vi "Process.vi"(8 "error in":errorcluster, 11 "TestDefaultDirectory In":refnum<class "Maui.Test.DefaultDirectory.lvclass">) -> (0 "error out":errorcluster, 3 "TestDefaultDirectory Out":refnum<class "Maui.Test.DefaultDirectory.lvclass">)   [LabVIEW 2019, in "Maui.Test.DefaultDirectory.lvclass"]
doc: "---------------------------------------------------------------\nJKI State Machine Objects™\nhttp://jki.net/state-machine-objects/\nCopyright (C) 2005-2015, JKI <info@jki.net>\nALL RIGHTS RESERVEDJKI State Machine Objects (SMO) 1.0.0.5\nJKI - JKI\nCopyright (c) 2016, JKI"
uses:
  Maui.Test.DefaultDirectory.lvclass
  C:/Program Files (x86)/National Instruments/LabVIEW 2019/vi.lib/JKI/JKI SMO/SMO/SMO.lvclass
  C:/Users/patrick/Documents/GitHub/MAUI-Engine/lvsrc/Maui 1.0/SMO.UI.MAUI/MAUI.lvclass
  C:/Program Files (x86)/National Instruments/LabVIEW 2019/vi.lib/JKI/JKI SMO/SMO.UI/SMO.UI.lvclass
  <vilib>/JKI/JKI SMO/SMO/Typedefs/Parent Call--Enum.ctl
  <userlib>/LevyLab/Embedded UI/SMO.UI.Embedded/Embedded UI.lvclass
  <vilib>/JKI/JKI SMO/SMO/SMO.lvclass/SMO.ctl
  Maui.Test.DefaultDirectory.lvclass/Maui.Test.DefaultDirectory.ctl
  lvsrc/Maui 1.0/SMO.UI.MAUI/Typedefs/PanelData.ctl
  <vilib>/JKI/JKI SMO/SMO/Private/ReftoDVR--SMO.vi
  <vilib>/addons/_JKI Toolkits/Caraya/classes/Assert/Assert True.vi
  <vilib>/addons/_JKI Toolkits/Caraya/classes/Assert/Assert Equal Value_Variant.vi
  lvsrc/Maui 1.0/SMO.UI.MAUI/MAUI.lvclass
  <vilib>/JKI/JKI SMO/SMO/SMO.lvclass
  <vilib>/JKI/JKI SMO/SMO.UI/SMO.UI.lvclass
  <vilib>/addons/_JKI Toolkits/Caraya/classes/Test/Test.lvclass
  <vilib>/addons/_JKI Toolkits/Caraya/classes/Assert/Assert.lvclass
panel:
  in  "Ring 2":u16(ring)
  in  "Ring 1":u16(ring)
  # "For instructions on how to use the JKI State Machine Objects, examples and video tutorials, visit:\nhttp://jki.net/state-machine-objects/\n\nJKI State Machine Objects™\nhttp://jki.net/state-machine-objects/\nCopyright (C) 2005-2015, JKI <info@jki.net>\nALL RIGHTS RESERVED"
  # "Test Default Directory"
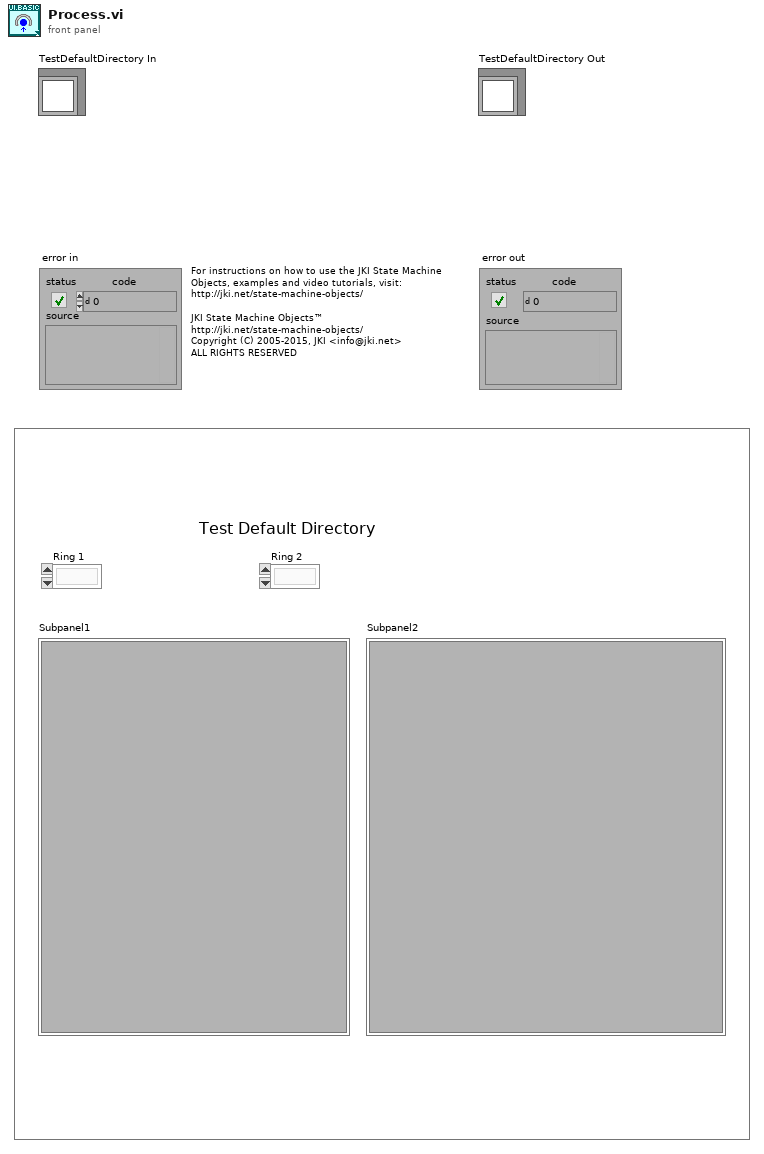
[diagram p1: front panel]
types:
  T1 = typedef "SMO.lvclass/Parent Call--Enum.ctl" = enum16{"Allows parent to run", "Does not request parent to run"}
  T2 = enum32{"invalid app kind", "Development System", "Run Time System", "Student Edition", "Embedded LabVIEW", "Evaluation", "Custom"}
  T3 = enum32{"Invalid", "Standard", "Closed", "Hidden", "Minimized", "Maximized"}
  T4 = cluster{"Core":cluster{"Current VI Reference":refnum<vi>, "Close Panel on Exit?":bool, "error":errorcluster}, "Self Reference":refnum<class "Maui.Test.DefaultDirectory.lvclass">, "Subpanel1":refnum<vi>, "Subpanel2":refnum<vi>, "Ring 1":refnum<vi>, "Ring 2":refnum<vi>, "Subpanels":refnum<class "Embedded UI.lvclass">[]}
  T5 = cluster{"Current VI Reference":refnum<vi>, "Close Panel on Exit?":bool, "error":errorcluster}
  T6 = typedef "SMO.lvclass/Protected Events.ctl" = cluster{"StopProcesses":refnum<user-event>, "AbortProcesses":refnum<user-event>, "Config Changed":refnum<user-event>, "Dependency":refnum<user-event>}
  T7 = typedef "MAUI.lvclass/PublicEvents--Cluster.ctl" = cluster{"ReadyForInfo ":refnum<user-event>}
  T8 = typedef "MAUI.lvclass/PanelData.ctl" = cluster{"SubPanel":refnum<vi>, "Ring":refnum<vi>, "Active":i32}
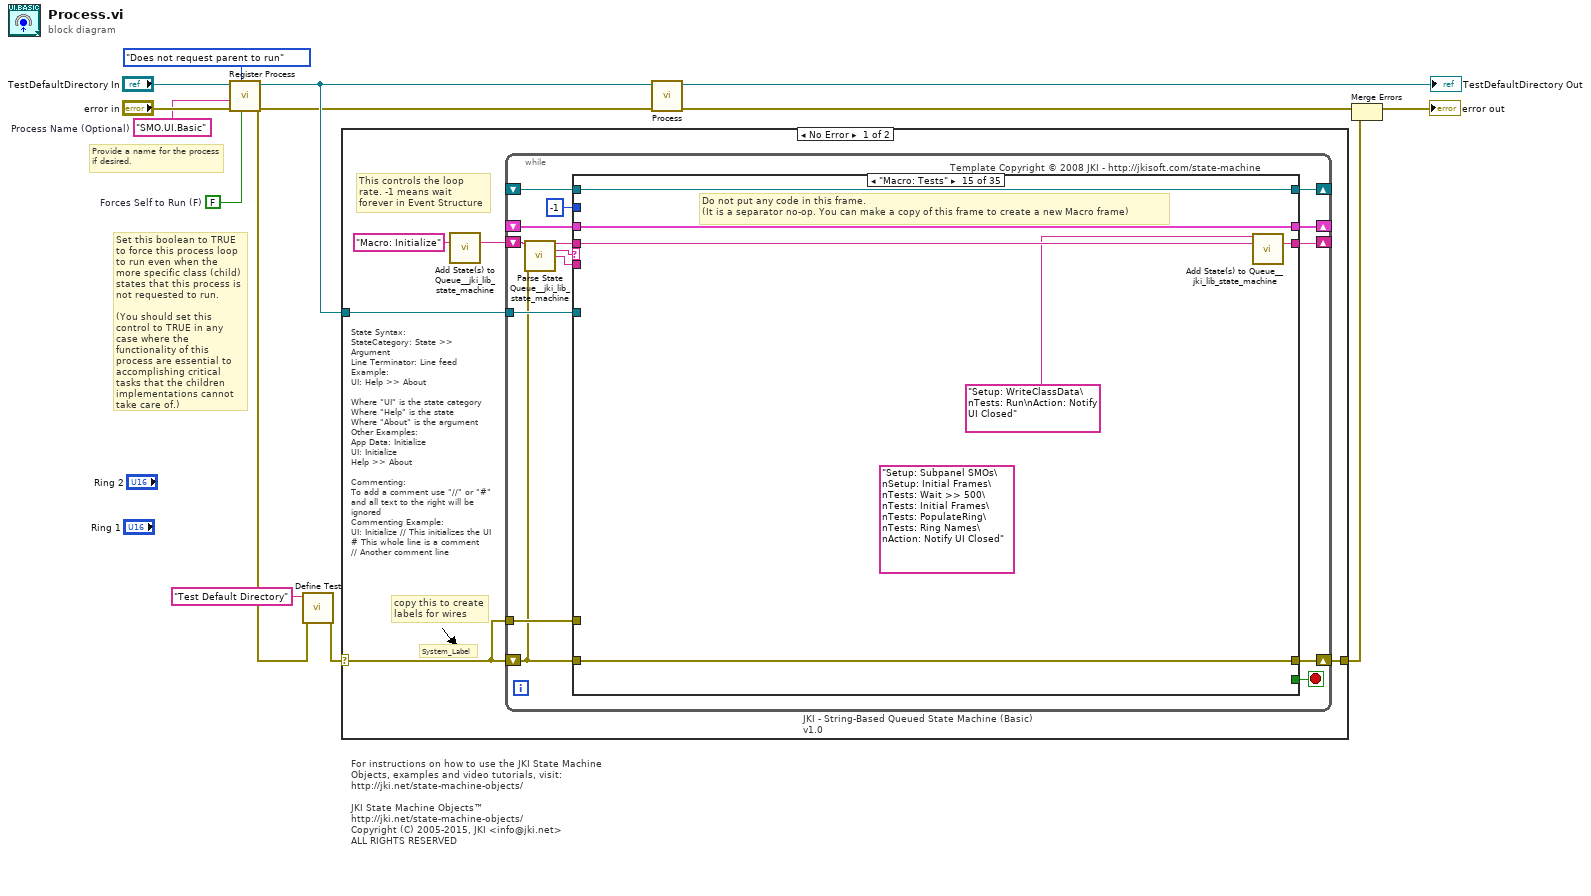
[diagram p0: block diagram]
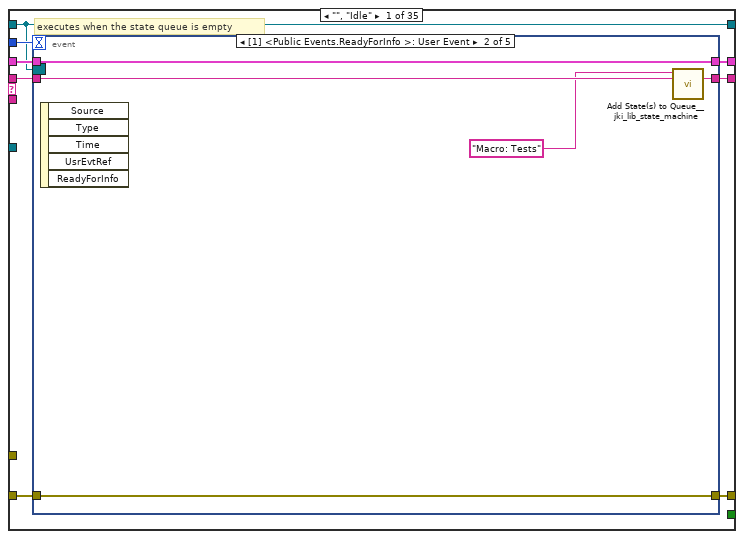
[diagram p2: hidden frame]
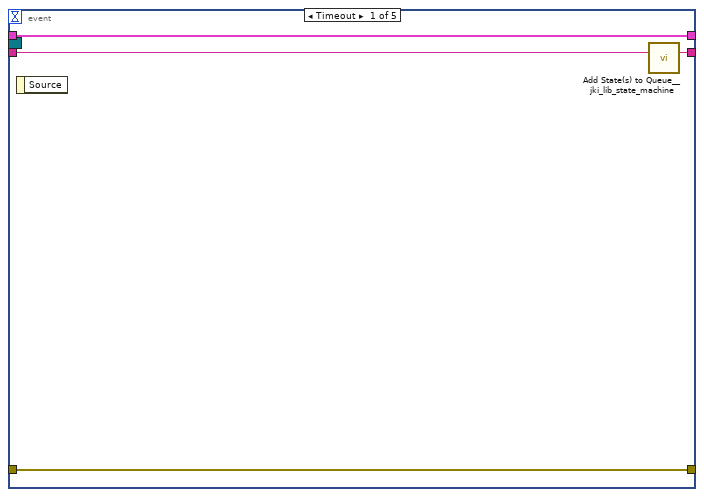
[diagram p3: hidden frame]
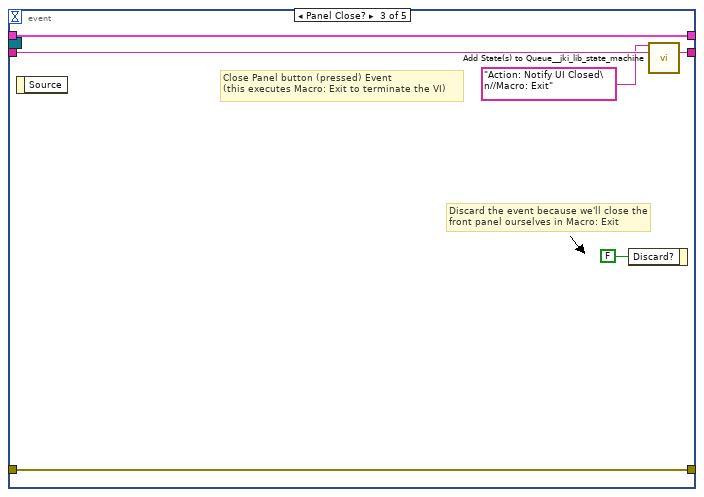
[diagram p4: hidden frame]
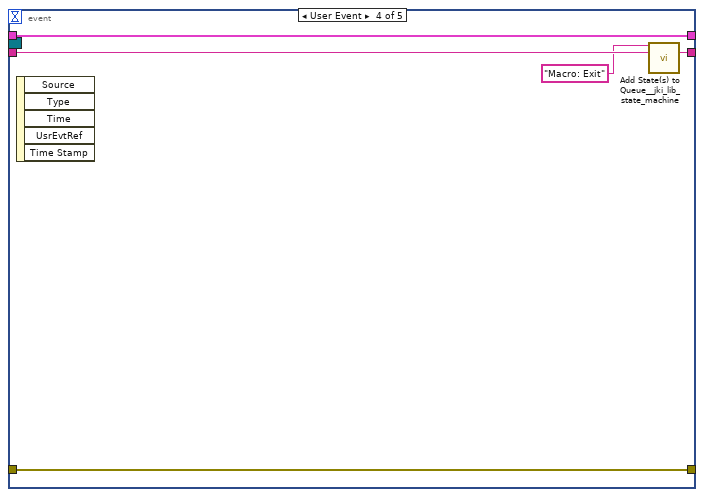
[diagram p5: hidden frame]
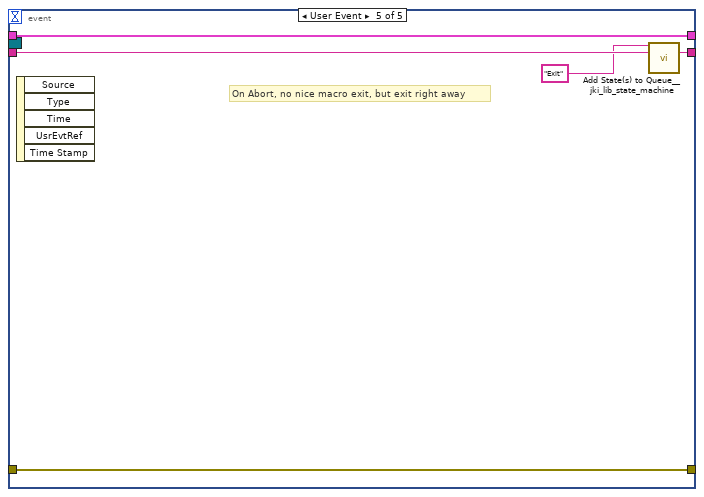
[diagram p6: hidden frame]
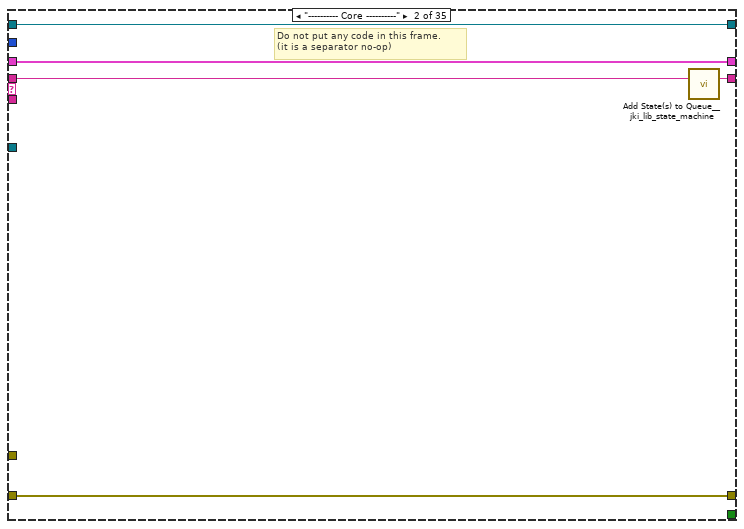
[diagram p7: hidden frame]
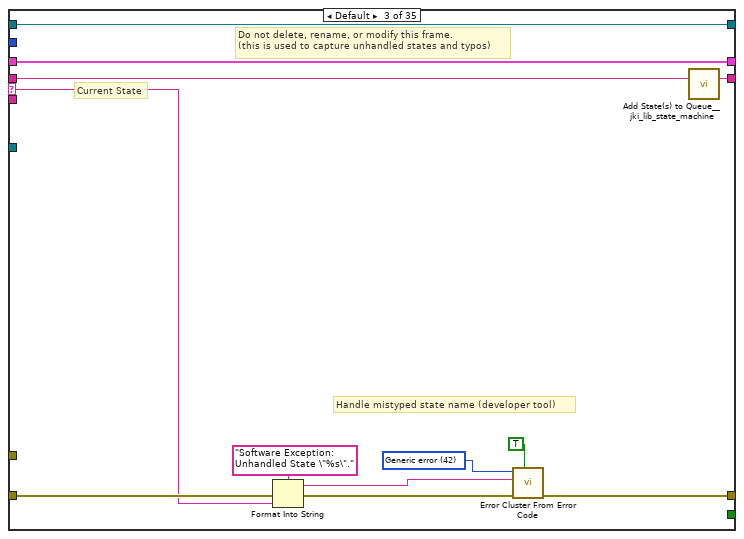
[diagram p8: hidden frame]
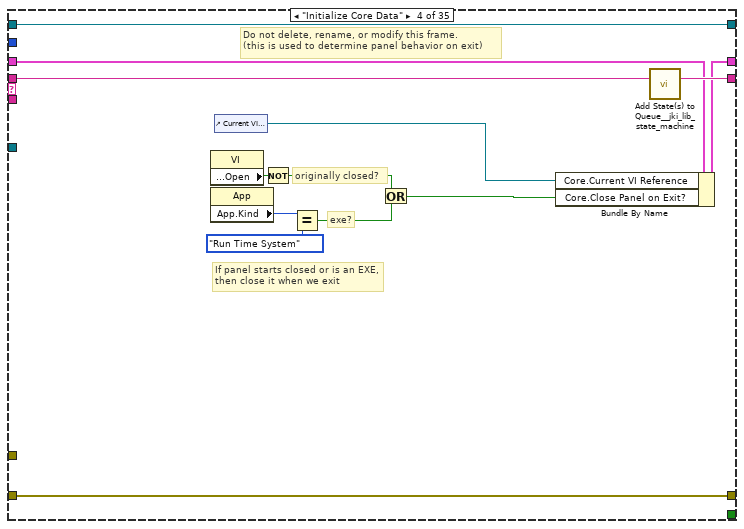
[diagram p9: hidden frame]
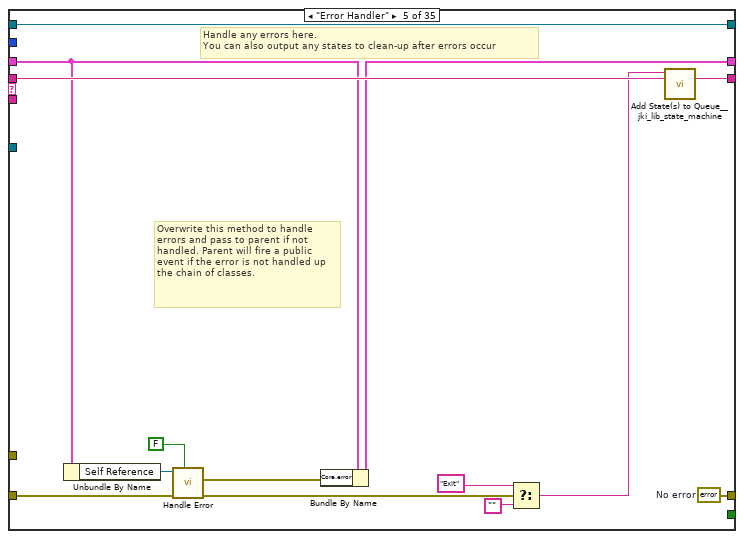
[diagram p10: hidden frame]
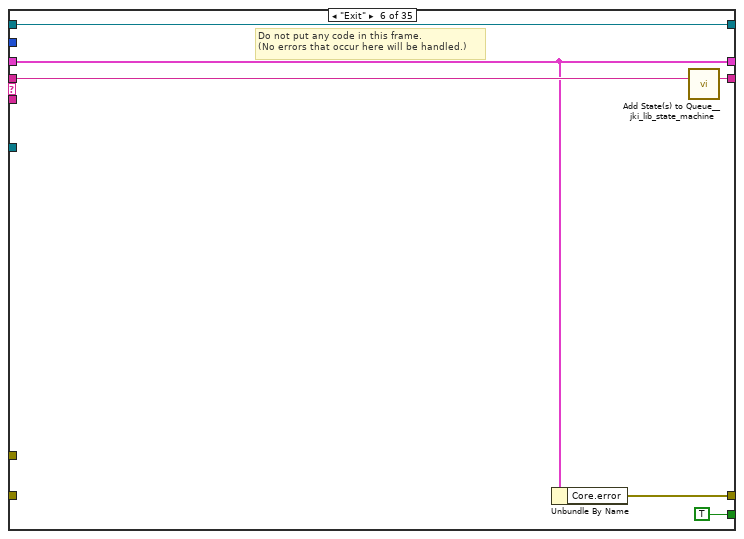
[diagram p11: hidden frame]
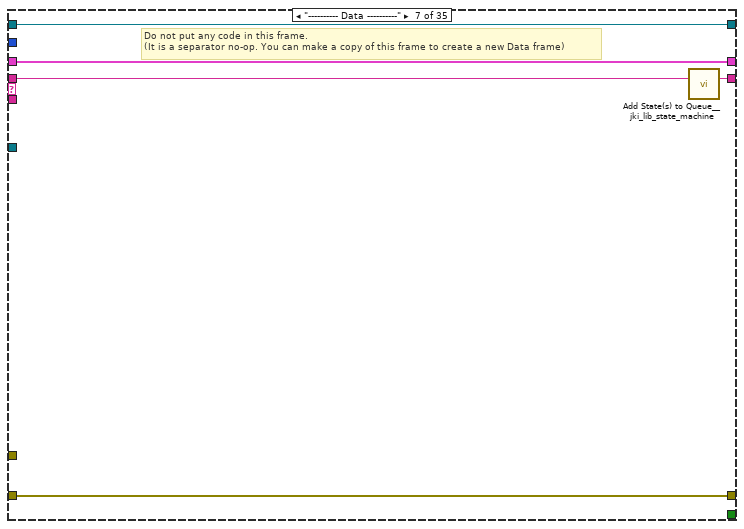
[diagram p12: hidden frame]
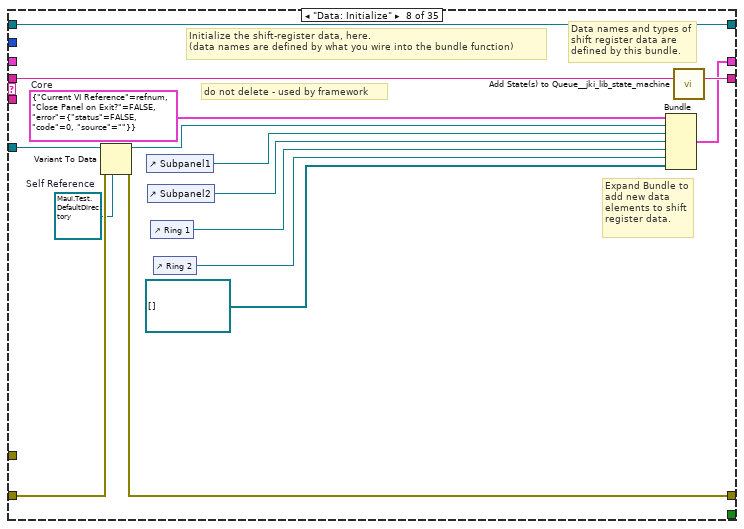
[diagram p13: hidden frame]
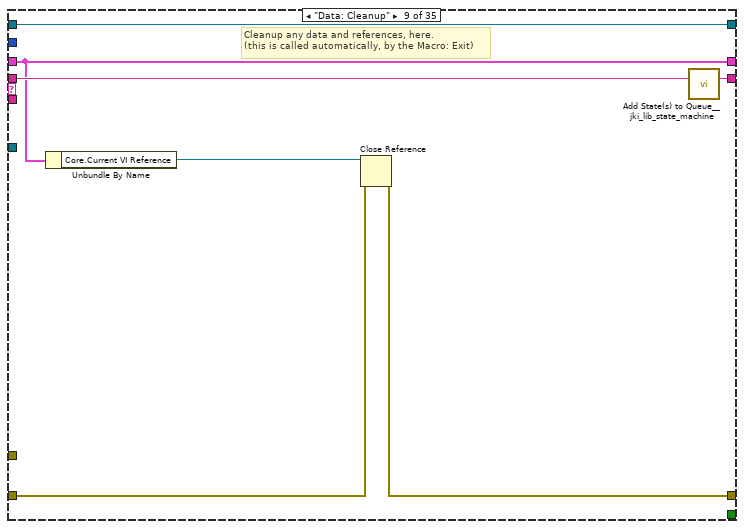
[diagram p14: hidden frame]
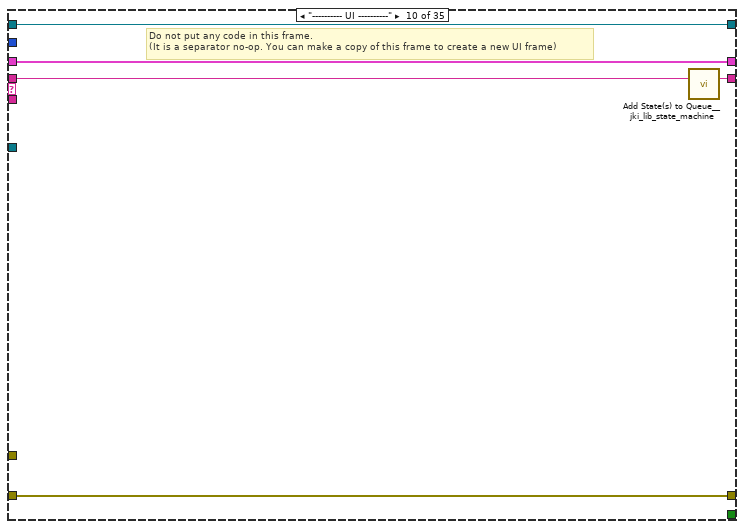
[diagram p15: hidden frame]
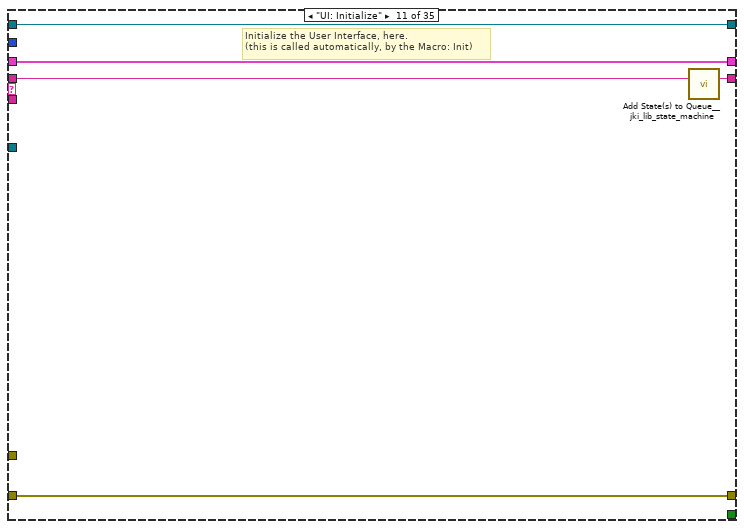
[diagram p16: hidden frame]
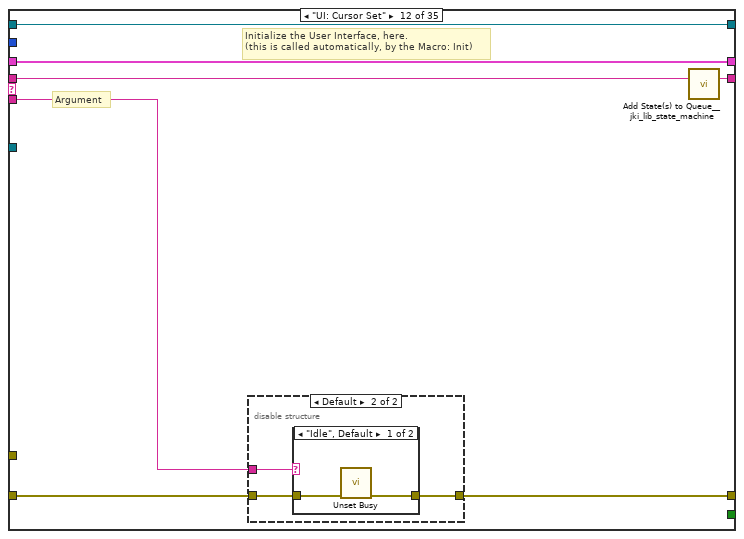
[diagram p17: hidden frame]
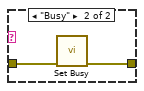
[diagram p19: hidden frame]
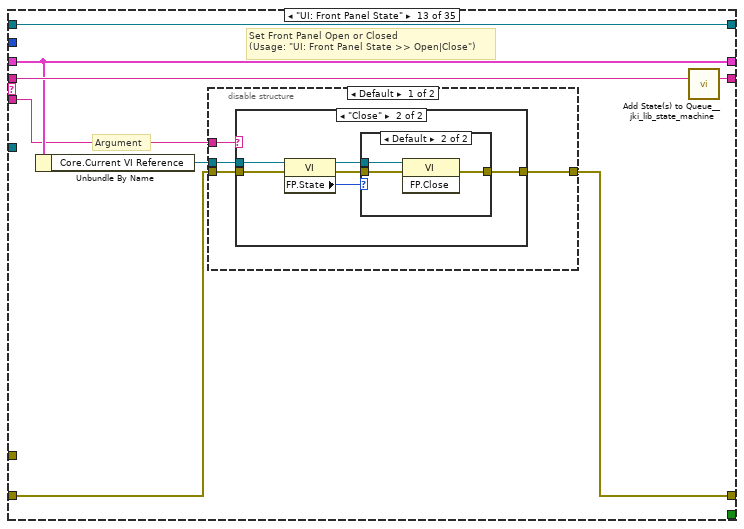
[diagram p20: hidden frame]
diagram:
  w5 = FALSE  # Forces Self to Run (F)
  w4 = "SMO.UI.Basic"  # Process Name (Optional)
  # "Provide a name for the process\nif desired."
  # "Set this boolean to TRUE to force this process loop to run even when the more specific class (child) states that this process is not requested to run.\n\n(You should set this control to TRUE in any case where the functionality of this process are essential to accomplishing critical tasks that the children implementations cannot take care of.)"
  # "For instructions on how to use the JKI State Machine Objects, examples and video tutorials, visit:\nhttp://jki.net/state-machine-objects/\n\nJKI State Machine Objects™\nhttp://jki.net/state-machine-objects/\nCopyright (C) 2005-2015, JKI <info@jki.net>\nALL RIGHTS RESERVED"
  n1 = call <vilib>:"Register Process.vi"("Forces Self to Run (F)"=w5, "Parent Call"=Parent_Call--Enum."Does not request parent to run", "error in (no error)"="error in", "Process Name (optional)"=w4, "SMO"="TestDefaultDirectory In") -> ("error out"=w3:errorcluster, "SMO out"=w10:refnum<class "Maui.Test.DefaultDirectory.lvclass">)  [unwired: 5 in]
  n2 = call <vilib>:"Define Test.vi"("error in (no error)"=w3, "Label (VI Title)"="Test Default Directory") -> ("error out"=w2:errorcluster)  [unwired: 9 in]
  n3 = case shown="No Error" w2 {
    selector: w2 -> [w15 w466]
    tunnel: w10 -> [w16 _]
    tunnel: [w14 w466] -> w7
    frame No Error {
      # "State Syntax:\nStateCategory: State >> Argument\nLine Terminator: Line feed\nExample:\nUI: Help >> About\n\nWhere \"UI\" is the state category\nWhere \"Help\" is the state\nWhere \"About\" is the argument\nOther Examples:\nApp Data: Initialize\nUI: Initialize\nHelp >> About\n\nCommenting:\nTo add a comment use \"//\" or \"#\" and all text to the right will be ignored\nCommenting Example:\nUI: Initialize // This initializes the UI\n# This whole line is a comment\n// Another comment line"
      # "copy this to create labels for wires"
      # "This controls the loop rate. -1 means wait forever in Event Structure"
      # "System_Label"
      n4 = call <vilib>:"Add State(s) to Queue__jki_lib_state_machine.vi"("State(s) in (\"\")"="Macro: Initialize") -> ("States Out"=w17:string)  [unwired: 14 in]
      n5 = while "JKI - String-Based Queued State Machine (Basic) v1.0" {
        shift-right: [w26] -> _
        shift-left: _ -> [w25]
        shift-right: [w29] -> w14
        shift-left: w15 -> [w19]
        shift-right: [w28] -> _
        shift-left: w17 -> [w30]
        tunnel: w16 -> [w23]
        shift-right: [w22] -> _
        shift-left: _ -> [w21]
        tunnel: w15 -> [w20]
        stop <- w27 stop-if-true
        # "Template Copyright © 2008 JKI - http://jkisoft.com/state-machine"
        n6 = call <vilib>:"Parse State Queue__jki_lib_state_machine.vi"("State Queue"=w30, "Error In (no error)"=w19) -> ("Remaining States"=w32:string, "Current State"=w33:string, "Arguments"=w31:string)  [unwired: 11 in]
        n7 = case shown="\"Macro: Tests\"" w33 {
          selector: w33 -> [_ _ w73 _ _ _ _ _ _ _ _ _ _ _ _ _ _ _ _ _ _ _ _ _ _ _ _ _ _ _ _ _ _ _ _]
          tunnel: w32 -> [w41 w71 w77 w96 w110 w116 w121 w136 w143 w148 w153 w160 w176 w208 w214 w223 w237 w242 w253 w258 w270 w276 w283 w290 w297 w309 w319 w338 w345 w359 w369 w398 w407 w427 w465]
          tunnel: w31 -> [_ _ _ _ _ _ _ _ _ _ _ w154 w170 _ _ _ _ _ _ _ _ _ _ _ _ _ _ _ _ _ _ _ w402 _ _]
          tunnel: w25 -> [w39 w68 w75 w87 w99 w112 w118 _ w138 w145 w151 w158 w172 w205 w211 w219 w228 w239 w250 w255 w268 w274 w279 w286 w293 w305 w316 w335 w341 w356 w366 w395 w403 w420 w460]
          tunnel: [w38 w69 w79 w93 w101 w111 w119 w132 w139 w146 w150 w155 w173 w206 w212 w221 w235 w240 w244 w256 w263 w271 w280 w284 w294 w306 w312 w331 w342 w347 w364 w390 w404 w421 w446] -> w29
          tunnel: w19 -> [w37 w69 w78 w93 w106 _ w119 w133 w140 w146 w150 w156 w174 w206 w212 w221 w235 w240 w245 w256 w265 w272 w280 w285 w294 w306 w311 w330 w342 w349 w362 w376 w400 w409 w445]
          tunnel: [w40 w70 w76 w95 w109 w115 w120 w135 w142 w147 w152 w159 w175 w207 w213 w222 w236 w241 w252 w257 w269 w275 w282 w289 w296 w308 w318 w337 w344 w358 w368 w397 w406 w426 w464] -> w28
          tunnel: [_ _ _ _ _ TRUE _ _ _ _ _ _ _ _ _ _ _ _ _ _ _ _ _ _ _ _ _ _ _ _ _ _ _ _ _] -> w27
          tunnel: [w36 w68 w75 w94 w98 w112 w118 w134 w138 w145 w151 w158 w172 w205 w211 w219 w228 w239 w250 w255 w268 w274 w278 w286 w292 w304 w315 w334 w340 w355 w365 w394 w403 w420 w460] -> w26
          tunnel: -1 ("Timeout") -> [w35 _ _ _ _ _ _ _ _ _ _ _ _ _ _ _ _ _ _ _ _ _ _ _ _ _ _ _ _ _ _ _ _ _ _]
          tunnel: w23 -> [_ _ _ _ _ _ _ w131 _ _ _ _ _ _ _ _ _ _ _ _ _ _ _ _ _ _ _ _ _ _ _ _ _ _ _]
          tunnel: [w34 w67 w72 w84 w108 w113 w117 w129 w137 w144 w149 w157 w169 w204 w210 w220 w229 w238 w251 w254 w267 w273 w281 w288 w295 w307 w317 w336 w343 w357 w367 w396 w405 w425 w463] -> w22
          tunnel: w21 -> [w34 w67 w72 w84 w108 w113 w117 w129 w137 w144 w149 w157 w169 w204 w210 w220 w229 w238 w251 w254 _ w273 w281 w288 w295 w307 w317 w336 w343 w357 w367 w396 w405 w425 w463]
          tunnel: w20 -> [_ _ _ _ _ _ _ _ _ _ _ _ _ _ _ _ _ _ _ _ _ _ _ _ _ _ _ _ _ w346 _ w375 _ w408 w431]
          frame "", "Idle" {
            # "executes when the state queue is empty"
            n8 = event shown="[1] <Public Events.ReadyForInfo >: User Event" {
              selector: w34 -> [_ _ _ _ _]
              dyn-events: _ -> [_ _ _ _ _]
              timeout: w35 -> [_ _ _ _ _]
              tunnel: w41 -> [w45 w50 w56 w61 w66]
              tunnel: [w44 w49 w55 w60 w65] -> w40
              tunnel: w39 -> [w42 w47 w52 w58 w63]
              tunnel: [w43 w48 w51 w59 w64] -> w38
              tunnel: w37 -> [w43 w48 w51 w59 w64]
              tunnel: [w42 w47 w52 w58 w63] -> w36
              event Timeout {
                n9 = event-data() -> ()  [unwired: 1 in, 1 out]
                n10 = call <vilib>:"Add State(s) to Queue__jki_lib_state_machine.vi"("State(s) in (\"\")"=w45) -> ("States Out"=w44:string)  [unwired: 14 in]
              }
              event User Event {
                n11 = event-data() -> ()  [unwired: 1 in, 5 out]
                n12 = call <vilib>:"Add State(s) to Queue__jki_lib_state_machine.vi"("State(s) in Front (\"\")"="Macro: Tests", "State(s) in (\"\")"=w50) -> ("States Out"=w49:string)  [unwired: 13 in]
              }
              event Panel Close? {
                # "Discard the event because we'll close the front panel ourselves in Macro: Exit"
                # "Close Panel button (pressed) Event\n(this executes Macro: Exit to terminate the VI)"
                n13 = event-data() -> ()  [unwired: 1 in, 1 out]
                n14 = event-data ("Event Filter Node")("Discard?"=FALSE) -> ()  [unwired: 1 in, 1 out]
                n15 = call <vilib>:"Add State(s) to Queue__jki_lib_state_machine.vi"("State(s) in Front (\"\")"="Action: Notify UI Closed\n//Macro: Exit", "State(s) in (\"\")"=w56) -> ("States Out"=w55:string)  [unwired: 13 in]
              }
              event User Event {
                n16 = event-data() -> ()  [unwired: 1 in, 5 out]
                n17 = call <vilib>:"Add State(s) to Queue__jki_lib_state_machine.vi"("State(s) in Front (\"\")"="Macro: Exit", "State(s) in (\"\")"=w61) -> ("States Out"=w60:string)  [unwired: 13 in]
              }
              event User Event {
                # "On Abort, no nice macro exit, but exit right away"
                n18 = event-data() -> ()  [unwired: 1 in, 5 out]
                n19 = call <vilib>:"Add State(s) to Queue__jki_lib_state_machine.vi"("State(s) in Front (\"\")"="Exit", "State(s) in (\"\")"=w66) -> ("States Out"=w65:string)  [unwired: 13 in]
              }
            }
          }
          frame "---------- Core ----------" {
            # "Do not put any code in this frame.\n(it is a separator no-op)"
            n20 = call <vilib>:"Add State(s) to Queue__jki_lib_state_machine.vi"("State(s) in (\"\")"=w71) -> ("States Out"=w70:string)  [unwired: 14 in]
          }
          frame Default {
            w82 = 42 items=["No error", "Argument error", "Memory is full", "Out of zone", "End of file", "File already open", "Generic file I/O error", "File not found", "File permission error", "Disk is full", "Duplicate path", "Too many files open", "System feature not enabled", "Resource file not found", "Cannot add resource", "Resource not found", "Image not found", "Image memory error", "Pen does not exist", "Config type invalid", "Config token not found", "Config parse error", "Config memory error", "Bad external code format", "Bad external code offset", "External code not present", "Null window", "Destroy window error", "Null menu", "Print aborted", "Bad print record", "Print driver error", "Windows error during printing", "Memory error during printing", "Print dialog error", "Generic print error", "Invalid device refnum", "Device not found", "Device parameter error", "Device unit error", "Cannot open device", "Device call aborted", "Generic error", "Cancelled by user", "Object ID too low", "Object ID too high", "Object not in heap", "Unknown heap", "Unknown object (invalid DefProc)", "Unknown object (DefProc not in table)", "Message out of range", "Invalid (null) method", "Unknown message", "Manager call not supported", "Bad address", "Network operation in progress", "Network operation timed out", "Connection is busy", "Network attribute not supported", "Network error", "Address in use", "System out of memory", "Connection aborted", "Connection refused", "Not connected", "Already connected", "Connection closed", "Initialization error (interapplication manager)", "Bad occurrence", "Wait on unbound occurrence handler", "Occurrence queue overflow", "Datalog type conflict", "Unused", "Unrecognized type (interapplication manager)", "Memory corrupt", "Failed to make temporary DLL", "Old CIN version", "Drag socket not found", "Failed to load drop-object", "Failed to register OLE object", "Failed to release OLE object", "Format specifier type mismatch", "Unknown format specifier", "Too few format specifiers", "Too many format specifiers", "Scan failed", "Newer CIN version", "Error converting to variant", "Runtime menu error", "Password tampered", "Variant attribute not found", "Incompatible variant data type", "Event data is not available", "Event Store is not present", "Occurrence is not found", "Event Queue is not created", "Event info is not available", "Refnum passed is NULL", "Error retrieving Class GUID", "Error retrieving CoClass GUID", "Error retrieving TypeLib GUID.", "Bad built application magic bytes.", "Specific driver is different from the specific driver associated with the Logical Name.", "There is no session opened to the class driver.", "Max Error", "MAX - Error with config objects", "MAX - Error loading configuration", "MAX - Group not supported"]
            # "Current State"
            # "Do not delete, rename, or modify this frame.\n(this is used to capture unhandled states and typos)"
            # "Handle mistyped state name (developer tool)"
            n21 = Format Into String(format string="Software Exception: Unhandled State \"%s\"." ("message"), error in=w78, w73) -> (resulting string=w81:string, error out=w80:errorcluster)  [unwired: 1 in]
            n22 = call <vilib>:"Error Cluster From Error Code.vi"("show call chain? (False)"=TRUE, "error in (no error)"=w80, "error message (\"\")"=w81, "error code (0)"=w82) -> ("error out"=w79:errorcluster)  [unwired: 5 in]
            n23 = call <vilib>:"Add State(s) to Queue__jki_lib_state_machine.vi"("State(s) in (\"\")"=w77) -> ("States Out"=w76:string)  [unwired: 14 in]
          }
          frame "Initialize Core Data" {
            # "Do not delete, rename, or modify this frame.\n(this is used to determine panel behavior on exit)"
            # "originally closed?"
            # "exe?"
            # "If panel starts closed or is an EXE, then close it when we exit"
            n24 = property on="Property Node" class="VI"() -> ("Front Panel.Open"=w92:bool)  [unwired: 2 in, 2 out]
            n25 = property on="Property Node" class="App"() -> ("App.Kind"=w91:T2)  [unwired: 2 in, 2 out]
            n26 = control-ref of="Current VI Reference"() -> (w85:refnum<vi>)
            n27 = Not(x=w92) -> (.not. x?=w89:bool)
            n28 = Equal?(x=w91, y=T2."Run Time System" ("Application:Kind")) -> (x = y?=w88:bool)
            n29 = Or(x=w89, y=w88) -> (x .or. y?=w86:bool)
            n30 = Bundle By Name(cluster=w87, "Core.Current VI Reference"=w85, "Core.Close Panel on Exit?"=w86) -> (w94:T4)
            n31 = call <vilib>:"Add State(s) to Queue__jki_lib_state_machine.vi"("State(s) in (\"\")"=w96) -> ("States Out"=w95:string)  [unwired: 14 in]
          }
          frame "Error Handler" {
            w101 = errorcluster {"status"=FALSE, "code"=0, "source"=""}  # No error
            # "Overwrite this method to handle errors and pass to parent if not handled. Parent will fire a public event if the error is not handled up the chain of classes."
            # "Handle any errors here.\nYou can also output any states to clean-up after errors occur"
            n32 = Unbundle By Name(w99) -> ("Self Reference"=w107:refnum<class "Maui.Test.DefaultDirectory.lvclass">)
            n33 = call-dynamic "Handle Error.vi"("Stop on Unhandled Error (T)"=FALSE, "error in"=w106, "SMO"=w107) -> ("handling error"=w102:errorcluster, "Unhandled error"=w100:errorcluster)  [unwired: 6 in, 1 out]
            n34 = Bundle By Name(cluster=w99, "Core.error"=w100) -> (w98:T4)
            n35 = Select(t="Exit", s=w102, f="") -> (s? t:f=w103:string)
            n36 = call <vilib>:"Add State(s) to Queue__jki_lib_state_machine.vi"("State(s) in Front (\"\")"=w103, "State(s) in (\"\")"=w110) -> ("States Out"=w109:string)  [unwired: 13 in]
          }
          frame "Exit" {
            # "Do not put any code in this frame.\n(No errors that occur here will be handled.)"
            n37 = Unbundle By Name(w112) -> ("Core.error"=w111:errorcluster)
            n38 = call <vilib>:"Add State(s) to Queue__jki_lib_state_machine.vi"("State(s) in (\"\")"=w116) -> ("States Out"=w115:string)  [unwired: 14 in]
          }
          frame "---------- Data ----------" {
            # "Do not put any code in this frame.\n(It is a separator no-op. You can make a copy of this frame to create a new Data frame)"
            n39 = call <vilib>:"Add State(s) to Queue__jki_lib_state_machine.vi"("State(s) in (\"\")"=w121) -> ("States Out"=w120:string)  [unwired: 14 in]
          }
          frame "Data: Initialize" {
            w125 = refnum<class "Maui.Test.DefaultDirectory.lvclass"> refnum  # Self Reference
            w128 = T5 {"Current VI Reference"=refnum, "Close Panel on Exit?"=FALSE, "error"={"status"=FALSE, "code"=0, "source"=""}}  # Core
            # "do not delete - used by framework"
            # "Expand Bundle to add new data elements to shift register data."
            # "Data names and types of shift register data are defined by this bundle."
            # "Initialize the shift-register data, here.\n(data names are defined by what you wire into the bundle function)"
            n40 = Variant To Data(error in=w133, type=w125, Variant=w131) -> (data=w130:refnum<class "Maui.Test.DefaultDirectory.lvclass">, error out=w132:errorcluster)
            n41 = control-ref of="Subpanel1"() -> (w126:refnum<vi>)
            n42 = control-ref of="Subpanel2"() -> (w124:refnum<vi>)
            n43 = control-ref of="Ring 1"() -> (w123:refnum<vi>)
            n44 = control-ref of="Ring 2"() -> (w122:refnum<vi>)
            n45 = Bundle("Core"=w128, "Self Reference"=w130, "Subpanel1"=w126, "Subpanel2"=w124, "Ring 1"=w123, "Ring 2"=w122, "Subpanels"=refnum<class "Embedded UI.lvclass">[] []) -> (w134:T4)  [unwired: 1 in]
            n46 = call <vilib>:"Add State(s) to Queue__jki_lib_state_machine.vi"("State(s) in (\"\")"=w136) -> ("States Out"=w135:string)  [unwired: 14 in]
          }
          frame "Data: Cleanup" {
            # "Cleanup any data and references, here.\n(this is called automatically, by the Macro: Exit)"
            n47 = Unbundle By Name(w138) -> ("Core.Current VI Reference"=w141:refnum<vi>)
            n48 = Close Reference(reference=w141, error in (no error)=w140) -> (error out=w139:errorcluster)
            n49 = call <vilib>:"Add State(s) to Queue__jki_lib_state_machine.vi"("State(s) in (\"\")"=w143) -> ("States Out"=w142:string)  [unwired: 14 in]
          }
          frame "---------- UI ----------" {
            # "Do not put any code in this frame.\n(It is a separator no-op. You can make a copy of this frame to create a new UI frame)"
            n50 = call <vilib>:"Add State(s) to Queue__jki_lib_state_machine.vi"("State(s) in (\"\")"=w148) -> ("States Out"=w147:string)  [unwired: 14 in]
          }
          frame "UI: Initialize" {
            # "Initialize the User Interface, here.\n(this is called automatically, by the Macro: Init)"
            n51 = call <vilib>:"Add State(s) to Queue__jki_lib_state_machine.vi"("State(s) in (\"\")"=w153) -> ("States Out"=w152:string)  [unwired: 14 in]
          }
          frame "UI: Cursor Set" {
            # "Argument"
            # "Initialize the User Interface, here.\n(this is called automatically, by the Macro: Init)"
            n52 = disable-structure "Conditional Disable Structure" shown="Default" {
              disable-tunnel: w156 -> [w161 w164]
              disable-tunnel: [w161 w163] -> w155
              disable-tunnel: w154 -> [_ w162]
              frame condition #0 {
              }
              frame condition #1 (active) {
                n53 = case shown="\"Idle\", Default" w162 {
                  tunnel: w164 -> [w166 w168]
                  tunnel: [w165 w167] -> w163
                  frame "Idle", Default {
                    n54 = call <vilib>:"Unset Busy.vi"("error in (no error)"=w166) -> ("error out"=w165:errorcluster)  [unwired: 10 in]
                  }
                  frame "Busy" {
                    n55 = call <vilib>:"Set Busy.vi"("error in (no error)"=w168) -> ("error out"=w167:errorcluster)  [unwired: 9 in, 1 out]
                  }
                }
              }
            }
            n56 = call <vilib>:"Add State(s) to Queue__jki_lib_state_machine.vi"("State(s) in (\"\")"=w160) -> ("States Out"=w159:string)  [unwired: 14 in]
          }
          frame "UI: Front Panel State" {
            # "Argument"
            # "Set Front Panel Open or Closed\n(Usage: \"UI: Front Panel State >> Open|Close\")"
            n57 = Unbundle By Name(w172) -> ("Core.Current VI Reference"=w171:refnum<vi>)
            n58 = disable-structure "Conditional Disable Structure" shown="Default" {
              disable-tunnel: w174 -> [w180 w203]
              disable-tunnel: [w179 w203] -> w173
              disable-tunnel: w171 -> [w178 _]
              disable-tunnel: w170 -> [w177 _]
              frame condition #0 (active) {
                n59 = case shown="\"Close\"" w177 {
                  tunnel: w180 -> [w184 w197]
                  tunnel: [w186 w198] -> w179
                  tunnel: w178 -> [w185 w195]
                  frame "Open", Default {
                    n60 = property on="Property Node" class="VI"(reference=w185, error in=w184) -> (reference out=w182:refnum<vi>, error out=w183:errorcluster, "FP.State"=w181:T3)
                    n61 = case shown="\"Closed\"" w181 {
                      tunnel: [w189 w192] -> w186
                      tunnel: w183 -> [w188 w192]
                      tunnel: w182 -> [w187 _]
                      frame "Closed" {
                        n62 = invoke on="Invoke Node" class="VI" method="FP.Open"(reference=w187, error in=w188, "Activate"=TRUE, "State"=T3."Standard") -> (error out=w189:errorcluster)  [unwired: 1 in, 4 out]
                      }
                      frame Default {
                      }
                    }
                  }
                  frame "Close" {
                    n63 = property on="Property Node" class="VI"(reference=w195, error in=w197) -> (reference out=w194:refnum<vi>, error out=w196:errorcluster, "FP.State"=w193:T3)
                    n64 = case shown="Default" w193 {
                      tunnel: [w199 w202] -> w198
                      tunnel: w196 -> [w199 w201]
                      tunnel: w194 -> [_ w200]
                      frame "Invalid", "Closed" {
                      }
                      frame Default {
                        n65 = invoke on="Invoke Node" class="VI" method="FP.Close"(reference=w200, error in=w201) -> (error out=w202:errorcluster)  [unwired: 1 in, 2 out]
                      }
                    }
                  }
                }
              }
              frame condition #1 {
              }
            }
            n66 = call <vilib>:"Add State(s) to Queue__jki_lib_state_machine.vi"("State(s) in (\"\")"=w176) -> ("States Out"=w175:string)  [unwired: 14 in]
          }
          frame "---------- Macro ----------" {
            # "Do not put any code in this frame.\n(It is a separator no-op. You can make a copy of this frame to create a new Macro frame)"
            n67 = call <vilib>:"Add State(s) to Queue__jki_lib_state_machine.vi"("State(s) in (\"\")"=w208) -> ("States Out"=w207:string)  [unwired: 14 in]
          }
          frame "Macro: Tests" {
            (unwired) "Setup: Subpanel SMOs\nSetup: Initial Frames\nTests: Wait >> 500\nTests: Initial Frames\nTests: PopulateRing\nTests: Ring Names\nAction: Notify UI Closed" ("State(s) in Front (\"\")")
            # "Do not put any code in this frame.\n(It is a separator no-op. You can make a copy of this frame to create a new Macro frame)"
            n68 = call <vilib>:"Add State(s) to Queue__jki_lib_state_machine.vi"("State(s) in Front (\"\")"="Setup: WriteClassData\nTests: Run\nAction: Notify UI Closed", "State(s) in (\"\")"=w214) -> ("States Out"=w213:string)  [unwired: 13 in]
          }
          frame "Macro: Initialize" {
            w217 = "UI: Initialize\n//UI: Front Panel State >> Open"  # UI: Initialize //UI: Front Panel State >> Open
            # "Initialization Macro\n(This is called once, when the VI starts)"
            n69 = call <vilib>:"Add State(s) to Queue__jki_lib_state_machine.vi"("State(s) in Front (\"\")"="Data: Initialize\nInitialize Core Data\nEvents: Register", "State(s) in (\"\")"="Process: Sync", "State(s) at Back (\"\")"=w217) -> ("States Out"=w216:string)  [unwired: 12 in]
            n70 = call <vilib>:"Add State(s) to Queue__jki_lib_state_machine.vi"("State(s) in Front (\"\")"=w216, "State(s) in (\"\")"=w223) -> ("States Out"=w222:string)  [unwired: 13 in]
          }
          frame "Macro: Exit" {
            # "Exit Macro\n(This is called once, when the VI exits)"
            n71 = Unbundle By Name(w228) -> ("Core.Close Panel on Exit?"=w234:bool)
            n72 = Select(t="//UI: Front Panel State >> Close", s=w234, f="") -> (s? t:f=w231:string)
            n73 = call <vilib>:"Add State(s) to Queue__jki_lib_state_machine.vi"("State(s) in Front (\"\")"="Data: Cleanup\nEvents: Unregister", "State(s) in (\"\")"="Process: Sync", "State(s) at Back (\"\")"="Exit") -> ("States Out"=w225:string)  [unwired: 12 in]
            n74 = call <vilib>:"Add State(s) to Queue__jki_lib_state_machine.vi"("State(s) in (\"\")"=w231, "State(s) at Back (\"\")"=w225) -> ("States Out"=w230:string)  [unwired: 13 in]
            n75 = call <vilib>:"Add State(s) to Queue__jki_lib_state_machine.vi"("State(s) in Front (\"\")"=w230, "State(s) in (\"\")"=w237) -> ("States Out"=w236:string)  [unwired: 13 in]
          }
          frame "---------- Process ----------" {
            # "Template Separator\n(You can make a copy of, or modify, this frame)"
            n76 = call <vilib>:"Add State(s) to Queue__jki_lib_state_machine.vi"("State(s) in (\"\")"=w242) -> ("States Out"=w241:string)  [unwired: 14 in]
          }
          frame "Process: Sync" {
            n77 = Unbundle By Name(w250) -> ("Self Reference"=w246:refnum<class "Maui.Test.DefaultDirectory.lvclass">)
            n78 = call <vilib>:"WaitOnProcessSync.vi"("error in (no error)"=w245, "SMO"=w246) -> ("error out"=w244:errorcluster, "Don't run?"=w249:bool)  [unwired: 7 in, 1 out]
            n79 = Select(t="Data: Cleanup\nEvents: Unregister\nExit", s=w249, f="") -> (s? t:f=w243:string)
            n80 = call <vilib>:"Add State(s) to Queue__jki_lib_state_machine.vi"("State(s) in Front (\"\")"=w243, "State(s) in (\"\")"=w253) -> ("States Out"=w252:string)  [unwired: 13 in]
          }
          frame "---------- Events ----------" {
            # "Template Separator\n(You can make a copy of, or modify, this frame)"
            n81 = call <vilib>:"Add State(s) to Queue__jki_lib_state_machine.vi"("State(s) in (\"\")"=w258) -> ("States Out"=w257:string)  [unwired: 14 in]
          }
          frame "Events: Register" {
            # "Expand to add\nmore events"
            # "Base Class Protected Events"
            n82 = Unbundle By Name(w268) -> ("Self Reference"=w259:refnum<class "Maui.Test.DefaultDirectory.lvclass">)
            n83 = call <vilib>:"GetProtectedEvents.vi"("SMO"=w259) -> ("error out"=w262:errorcluster, "SMO Protected Events"=w266:T6)  [unwired: 8 in, 1 out]
            n84 = call "MAUI.GetPublicEvents.vi"("MAUI"=w259) -> ("error out"=w260:errorcluster, "Public Events"=w261:T7)  [unwired: 8 in, 1 out]
            n85 = register-events(w266, w261) -> (reference out=w267:refnum<event-registration>, error out=w264:errorcluster)  [unwired: 2 in]
            n86 = Merge Errors(w260, w265, w264, w262) -> (w263:errorcluster)
            n87 = call <vilib>:"Add State(s) to Queue__jki_lib_state_machine.vi"("State(s) in (\"\")"=w270) -> ("States Out"=w269:string)  [unwired: 14 in]
          }
          frame "Events: Unregister" {
            n88 = Unregister For Events(event registration refnum=w273, error in=w272) -> (error out=w271:errorcluster)
            n89 = call <vilib>:"Add State(s) to Queue__jki_lib_state_machine.vi"("State(s) in (\"\")"=w276) -> ("States Out"=w275:string)  [unwired: 14 in]
          }
          frame "---------- Action ----------" {
            n90 = Unbundle By Name(w279) -> ("Self Reference"=w277:refnum<class "Maui.Test.DefaultDirectory.lvclass">)
            n91 = Bundle By Name(cluster=w279, "Self Reference"=w277) -> (w278:T4)
            n92 = call <vilib>:"Add State(s) to Queue__jki_lib_state_machine.vi"("State(s) in (\"\")"=w283) -> ("States Out"=w282:string)  [unwired: 14 in]
          }
          frame "Action: Notify UI Closed" {
            # "Notify that the UI has been closed"
            n93 = Unbundle By Name(w286) -> ("Self Reference"=w287:refnum<class "Maui.Test.DefaultDirectory.lvclass">)
            n94 = call <vilib>:"Hide.vi"("error in (no error)"=w285, "SMO.UI"=w287) -> ("error out"=w284:errorcluster)  [unwired: 8 in, 1 out]
            n95 = call <vilib>:"Add State(s) to Queue__jki_lib_state_machine.vi"("State(s) in (\"\")"=w290) -> ("States Out"=w289:string)  [unwired: 14 in]
          }
          frame "---------- Setup ----------" {
            n96 = Unbundle By Name(w293) -> ("Self Reference"=w291:refnum<class "Maui.Test.DefaultDirectory.lvclass">)
            n97 = Bundle By Name(cluster=w293, "Self Reference"=w291) -> (w292:T4)
            n98 = call <vilib>:"Add State(s) to Queue__jki_lib_state_machine.vi"("State(s) in (\"\")"=w297) -> ("States Out"=w296:string)  [unwired: 14 in]
          }
          frame "Setup: WriteClassData" {
            n99 = Unbundle By Name(w305) -> ("Self Reference"=w303:refnum<class "Maui.Test.DefaultDirectory.lvclass">, "Subpanel1"=w301:refnum<vi>, "Ring 1"=w300:refnum<vi>, "Subpanel2"=w299:refnum<vi>, "Ring 2"=w298:refnum<vi>)
            n100 = Bundle By Name(cluster=w303, "Panel 1"=w301, "Ring 1"=w300, "Panel 2"=w299, "Ring 2"=w298) -> (w302:refnum<class "Maui.Test.DefaultDirectory.lvclass">)
            n101 = Bundle By Name(cluster=w305, "Self Reference"=w302) -> (w304:T4)
            n102 = call <vilib>:"Add State(s) to Queue__jki_lib_state_machine.vi"("State(s) in (\"\")"=w309) -> ("States Out"=w308:string)  [unwired: 14 in]
          }
          frame "Setup: Subpanel SMOs" {
            n103 = Unbundle By Name(w316) -> ("Self Reference"=w314:refnum<class "Maui.Test.DefaultDirectory.lvclass">)
            n104 = call "ReadEmbedded.vi"("error in (no error)"=w311, "MAUI in"=w314) -> ("error out"=w312:errorcluster, "Subpanels"=w310:refnum<class "Embedded UI.lvclass">[], "MAUI out"=w313:refnum<class "Maui.Test.DefaultDirectory.lvclass">)  [unwired: 7 in]
            n105 = Bundle By Name(cluster=w316, "Self Reference"=w313, "Subpanels"=w310) -> (w315:T4)
            n106 = call <vilib>:"Add State(s) to Queue__jki_lib_state_machine.vi"("State(s) in (\"\")"=w319) -> ("States Out"=w318:string)  [unwired: 14 in]
          }
          frame "Setup: Initial Frames" {
            w329 = T8 {"SubPanel"=refnum, "Ring"=refnum, "Active"=0} ("Panel")
            # "What happens in the init sequence that I need to test?"
            n107 = Unbundle By Name(w335) -> ("Self Reference"=w333:refnum<class "Maui.Test.DefaultDirectory.lvclass">, "Subpanel1"=w328:refnum<vi>, "Ring 1"=w327:refnum<vi>, "Subpanel2"=w326:refnum<vi>, "Ring 2"=w325:refnum<vi>)
            n108 = Bundle(cluster=w329, "SubPanel"=w328, "Ring"=w327, "Active"=0) -> (w324:T8)
            n109 = Bundle(cluster=w329, "SubPanel"=w326, "Ring"=w325, "Active"=1) -> (w323:T8)
            n110 = Build Array(w324, w323) -> (w322:T8[])
            n111 = call "WritePanelData.vi"("error in (no error)"=w330, "Panel Data Array"=w322, "MAUI in"=w333) -> ("error out"=w331:errorcluster, "MAUI out"=w332:refnum<class "Maui.Test.DefaultDirectory.lvclass">)  [unwired: 7 in]
            n112 = Bundle By Name(cluster=w335, "Self Reference"=w332) -> (w334:T4)
            n113 = call <vilib>:"Add State(s) to Queue__jki_lib_state_machine.vi"("State(s) in (\"\")"=w338) -> ("States Out"=w337:string)  [unwired: 14 in]
          }
          frame "Setup: Change Frames" {
            n114 = Unbundle By Name(w341) -> ("Self Reference"=w339:refnum<class "Maui.Test.DefaultDirectory.lvclass">)
            n115 = Bundle By Name(cluster=w341, "Self Reference"=w339) -> (w340:T4)
            n116 = call <vilib>:"Add State(s) to Queue__jki_lib_state_machine.vi"("State(s) in (\"\")"=w345) -> ("States Out"=w344:string)  [unwired: 14 in]
          }
          frame "---------- Tests ----------" {
            # "For Parallel tests:"
            n117 = Unbundle By Name(w356) -> ("Self Reference"=w354:refnum<class "Maui.Test.DefaultDirectory.lvclass">)
            n118 = call <vilib>:"Define Test.vi"("error in (no error)"=w346, "Label (VI Title)"="FrameTest") -> ("error out"=w350:errorcluster)  [unwired: 9 in]
            n119 = Bundle By Name(cluster=w356, "Self Reference"=w354) -> (w355:T4)
            n120 = call-poly <vilib>:"Assert.vi"("Label"="AssertionLabel" ("Label (VI Title)"), "error in (no error)"=w350, "True?"=TRUE) -> ("error out"=w351:errorcluster)  [unwired: 8 in]
            n121 = call <vilib>:"Add State(s) to Queue__jki_lib_state_machine.vi"("State(s) in (\"\")"=w359) -> ("States Out"=w358:string)  [unwired: 14 in]
            n122 = Merge Errors(w351, w349) -> (w347:errorcluster)
          }
          frame "Tests: Run" {
            n123 = Unbundle By Name(w366) -> ("Self Reference"=w361:refnum<class "Maui.Test.DefaultDirectory.lvclass">)
            n124 = call "Maui.Test.DefaultDirectory.RunAllTests.vi"("error in (no error)"=w362, "TestDefaultDirectory in"=w361) -> ("error out"=w363:errorcluster, "TestDefaultDirectory out"=w360:refnum<class "Maui.Test.DefaultDirectory.lvclass">)  [unwired: 8 in]
            n125 = Bundle By Name(cluster=w366, "Self Reference"=w360) -> (w365:T4)
            n126 = call <vilib>:"Add State(s) to Queue__jki_lib_state_machine.vi"("State(s) in (\"\")"=w369) -> ("States Out"=w368:string)  [unwired: 14 in]
            n127 = Merge Errors(w363) -> (w364:errorcluster)
          }
          frame "Tests: Ring Names" {
            # "For Parallel tests:"
            n128 = Unbundle By Name(w395) -> ("Self Reference"=w389:refnum<class "Maui.Test.DefaultDirectory.lvclass">, "Subpanels"=w384:refnum<class "Embedded UI.lvclass">[], "Ring 1"=w381:refnum<vi>, "Ring 2"=w380:refnum<vi>)
            n129 = call <vilib>:"Define Test.vi"("error in (no error)"=w375, "Label (VI Title)"="FrameTest") -> ("error out"=w374:errorcluster)  [unwired: 9 in]
            n130 = call <vilib>:"Get LV Class Path.vi"("object"=w389) -> ("class path"=w388:path)  [unwired: 9 in, 1 out]
            n131 = property on="Property Node" class="Ring (strict)"(reference=w381) -> ("Strings []"=w378:string[])  [unwired: 1 in, 2 out]
            n132 = property on="Property Node" class="Ring (strict)"(reference=w380) -> ("Strings []"=w371:string[])  [unwired: 1 in, 2 out]
            n133 = Array Size(array=w384) -> (size(s)=w370:i32)
            n134 = Strip Path(path=w388) -> (stripped path=w387:path)  [unwired: 1 out]
            n135 = Build Path(base path=w387, name or relative path="Subpanels") -> (appended path=w383:path)
            n136 = List Folder(path=w383) -> (folder names=w377:string[])  [unwired: 3 in, 3 out]
            n137 = Array Size(array=w377) -> (size(s)=w382:i32)
            n138 = Bundle By Name(cluster=w395, "Self Reference"=w389) -> (w394:T4)
            n139 = call-poly <vilib>:"Assert.vi"("Label"="Correct Number?" ("Label (VI Title)"), "error in (no error)"=w374, "Y"=w370, "X"=w382) -> ("error out"=w372:errorcluster)  [unwired: 7 in]
            n140 = call-poly <vilib>:"Assert.vi"("Label"="Ring 1: Strings are equal to subpanel class names located in folder" ("Label (VI Title)"), "error in (no error)"=w374, "Y"=w377, "X"=w378) -> ("error out"=w373:errorcluster)  [unwired: 7 in]
            n141 = call-poly <vilib>:"Assert.vi"("Label"="Ring 2: Strings are equal to subpanel class names located in folder" ("Label (VI Title)"), "error in (no error)"=w374, "Y"=w371, "X"=w377) -> ("error out"=w392:errorcluster)  [unwired: 7 in]
            n142 = call <vilib>:"Add State(s) to Queue__jki_lib_state_machine.vi"("State(s) in (\"\")"=w398) -> ("States Out"=w397:string)  [unwired: 14 in]
            n143 = Merge Errors(w372, w373, w392, w376) -> (w390:errorcluster)
          }
          frame "Tests: Wait" {
            n144 = Decimal String To Number(string=w402) -> (number=w399:i32)  [unwired: 2 in, 1 out]
            n145 = call <userlib>:"Wait (ms)__ogtk.vi"("error in (no error)"=w400, "milliseconds to wait"=w399) -> ("error out"=w401:errorcluster)  [unwired: 8 in, 1 out]
            n146 = call <vilib>:"Add State(s) to Queue__jki_lib_state_machine.vi"("State(s) in (\"\")"=w407) -> ("States Out"=w406:string)  [unwired: 14 in]
            n147 = Merge Errors(w401) -> (w404:errorcluster)
          }
          frame "Tests: PopulateRing" {
            # "For Parallel tests:"
            n148 = Unbundle By Name(w420) -> ("Subpanels"=w419:refnum<class "Embedded UI.lvclass">[], "Ring 1"=w418:refnum<vi>, "Ring 2"=w417:refnum<vi>)
            n149 = call <vilib>:"Define Test.vi"("error in (no error)"=w408, "Label (VI Title)"="Test Populate Rings") -> ("error out"=w414:errorcluster)  [unwired: 9 in]
            n150 = property on="Property Node" class="Ring (strict)"(reference=w418, error in=w414) -> (error out=w412:errorcluster, "Strings []"=w415:string[])  [unwired: 1 out]
            n151 = property on="Property Node" class="Ring (strict)"(reference=w417, error in=w414) -> (error out=w413:errorcluster, "Strings []"=w410:string[])  [unwired: 1 out]
            n152 = for {
              tunnel: w419 -> [w430] mode=indexing
              tunnel: [w429] -> w411 mode=indexing
              n153 = call <userlib>:"GetEmbeddedName.vi"("timeout in ms (-1)"=100, "EmbeddedSMO in"=w430) -> ("Name"=w429:string)  [unwired: 7 in, 2 out]
            }
            n154 = call-poly <vilib>:"Assert.vi"("Label"="Ring 1 Strings Are Correct" ("Label (VI Title)"), "error in (no error)"=w412, "Y"=w415, "X"=w411) -> ()  [unwired: 7 in, 1 out]
            n155 = call-poly <vilib>:"Assert.vi"("Label"="Ring 2 Strings Are Correct" ("Label (VI Title)"), "error in (no error)"=w413, "Y"=w411, "X"=w410) -> ("error out"=w423:errorcluster)  [unwired: 7 in]
            n156 = call <vilib>:"Add State(s) to Queue__jki_lib_state_machine.vi"("State(s) in (\"\")"=w427) -> ("States Out"=w426:string)  [unwired: 14 in]
            n157 = Merge Errors(w423, w409) -> (w421:errorcluster)
          }
          frame "Tests: Initial Frames" {
            w449 = 500 ("timeout in ms (-1)")
            n158 = Unbundle By Name(w460) -> ("Subpanels"=w459:refnum<class "Embedded UI.lvclass">[], "Subpanel1"=w450:refnum<vi>, "Subpanel2"=w447:refnum<vi>, "Ring 1"=w444:refnum<vi>, "Ring 2"=w438:refnum<vi>)
            n159 = call <vilib>:"Define Test.vi"("error in (no error)"=w431, "Label (VI Title)"="Test Initial Frame Action") -> ("error out"=w437:errorcluster)  [unwired: 9 in]
            n160 = Index Array(array=w459) -> (element #1=w455:refnum<class "Embedded UI.lvclass">, element #2=w454:refnum<class "Embedded UI.lvclass">)  [unwired: 2 in]
            n161 = property on="Property Node" class="Ring (strict)"(reference=w444, error in=w437) -> (error out=w440:errorcluster, "Disabled Items []"=w442:i32[])  [unwired: 1 out]
            n162 = property on="Property Node" class="Ring (strict)"(reference=w438, error in=w437) -> (error out=w436:errorcluster, "Disabled Items []"=w433:i32[])  [unwired: 1 out]
            n163 = call <userlib>:"GetSubPanelRef.vi"("timeout in ms (-1)"=w449, "error in (no error)"=w437, "EmbeddedSMO in"=w455) -> ("error out"=w452:errorcluster, "SubPanelReference"=w451:refnum<vi>)  [unwired: 6 in, 1 out]
            n164 = call <userlib>:"GetSubPanelRef.vi"("timeout in ms (-1)"=w449, "error in (no error)"=w437, "EmbeddedSMO in"=w454) -> ("error out"=w453:errorcluster, "SubPanelReference"=w448:refnum<vi>)  [unwired: 6 in, 1 out]
            n165 = call-poly <vilib>:"Assert.vi"("Label"="Panel 1 is correct", "error in (no error)"=w452, "Y"=w451, "X"=w450) -> ("error out"=w458:errorcluster)  [unwired: 7 in]
            n166 = call-poly <vilib>:"Assert.vi"("Label"="Panel 2 is Correct", "error in (no error)"=w453, "Y"=w448, "X"=w447) -> ("error out"=w462:errorcluster)  [unwired: 7 in]
            n167 = call-poly <vilib>:"Assert.vi"("Label"="Ring 1 Disabled Correctly", "error in (no error)"=w440, "Y"=i32[] [1] ("Disabled Items []"), "X"=w442) -> ("error out"=w439:errorcluster)  [unwired: 7 in]
            n168 = call-poly <vilib>:"Assert.vi"("Label"="Ring 1 Disabled Correctly", "error in (no error)"=w436, "Y"=i32[] [0] ("Disabled Items []"), "X"=w433) -> ("error out"=w435:errorcluster)  [unwired: 7 in]
            n169 = call <vilib>:"Add State(s) to Queue__jki_lib_state_machine.vi"("State(s) in (\"\")"=w465) -> ("States Out"=w464:string)  [unwired: 14 in]
            n170 = Merge Errors(w435, w439, w458, w462, w445) -> (w446:errorcluster)
          }
        }
      }
    }
    frame Error {
    }
  }
  n171 = call-parent "Process.vi"("error in"=w3, "MAUI"=w10) -> ("error out"=w8:errorcluster, "MAUI out"=→"TestDefaultDirectory Out":refnum<class "Maui.Test.DefaultDirectory.lvclass">)  [unwired: 8 in]
  n172 = Merge Errors(w8, w7) -> (→"error out":errorcluster)
